vi "lab2_question3.vi"() -> ()   [LabVIEW 2019]
uses:
  <vilib>/Platform/TimedLoop/XDataNode/timing_clust.ctl
  <vilib>/Platform/TimedLoop/XDataNode/nitl_modes.ctl
  <vilib>/Platform/TimedLoop/XDataNode/wakeup.ctl
  <vilib>/Analysis/3filter.llb/Filter Passband Type.ctl
  <vilib>/DAQmx/read.llb/DAQmx Read (Analog DBL 1Chan 1Samp).vi
  <vilib>/DAQmx/create/channels.llb/DAQmx Create Channel (AI-Voltage-Basic).vi
  <vilib>/DAQmx/miscellaneous.llb/DAQmx Fill In Error Info.vi
  <vilib>/platform/TimedLoop/XDataNode/XDataNode.xnode
  <vilib>/Platform/TimedLoop/XDataNode/XDNodeRunTimeDep.lvlib
  <vilib>/ptbypt/NI_PtbyPt.lvlib
  <vilib>/Analysis/NI_AALBase.lvlib
panel:
  out "Position [deg]":dbl(knob) scale=-32.5..32.5
  out "Iteration":i32
  in  "stop":bool
  out "Filtered Signal [V]":dbl
  out "Filtered Signal [V]":dbl(graph)
  in  "low cutoff freq: fl 2":dbl=0.125 format="%0.3f"
  out "Raw Signal [V]":dbl(graph)
  out "Raw Signal [V]":dbl
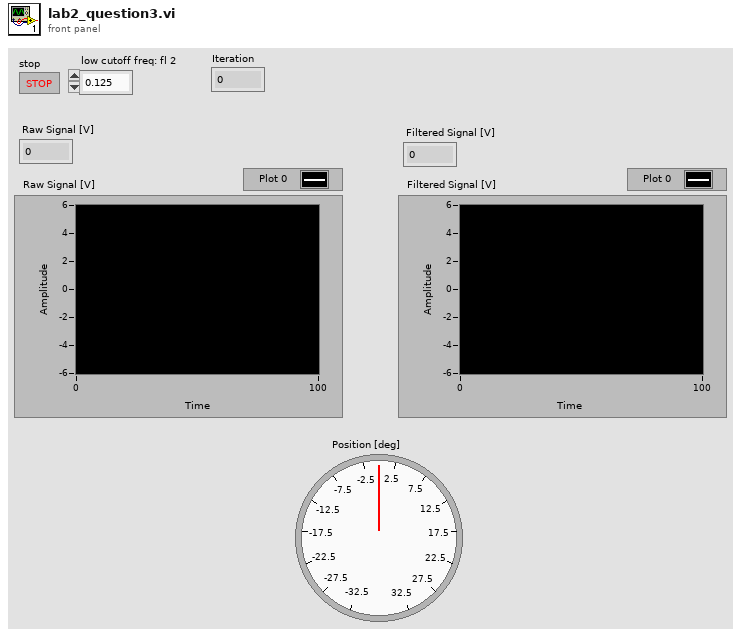
[diagram p1: front panel]
types:
  T1 = typedef "NI_AALBase.lvlib/Filter Passband Type.ctl" = enum32{"Lowpass", "Highpass", "Bandpass", "Bandstop"}
  T2 = typedef "XDNodeRunTimeDep.lvlib/timing_clust.ctl" = cluster{"Expected End [f-1]":u64, "Actual End [f-1]":u64, "Finished Late? [f-1]":bool, "Expected End [i-1]":u64, "Actual End [i-1]":u64, "Finished Late? [i-1]":bool, "Expected Start [i]":u64, "Actual Start [i]":u64, "Expected Start [f]":u64, "Actual Start [f]":u64, "Source Name":string, "Structure Name":string, "Period":i64, "Deadline":i64, "Offset":i64, "Start":i64, "Priority":i32, "Timeout":i32, "Mode":T3, "Wakeup Reason":T4, "Error":errorcluster, "Source Type":string, "Secondary Source Type":string, "Global End Time":u64, "Global Start Time":u64, "Frame Duration":u64, "Iteration Duration":u64, "Assigned CPU":i32, "I/O Scan Engine Mode":u32}
  T3 = typedef "XDNodeRunTimeDep.lvlib/nitl_modes.ctl" = enum32{"No Change", "Process missed periods, maintain original phase", "Discard missed periods, maintain original phase", "Process missed periods, ignore original phase", "Discard missed periods, ignore original phase"}
  T4 = typedef "XDNodeRunTimeDep.lvlib/wakeup.ctl" = enum32{"Normal", "Aborted", "Asynchronous wakeup", "Timing source error", "Timed loop error", "Timeout"}
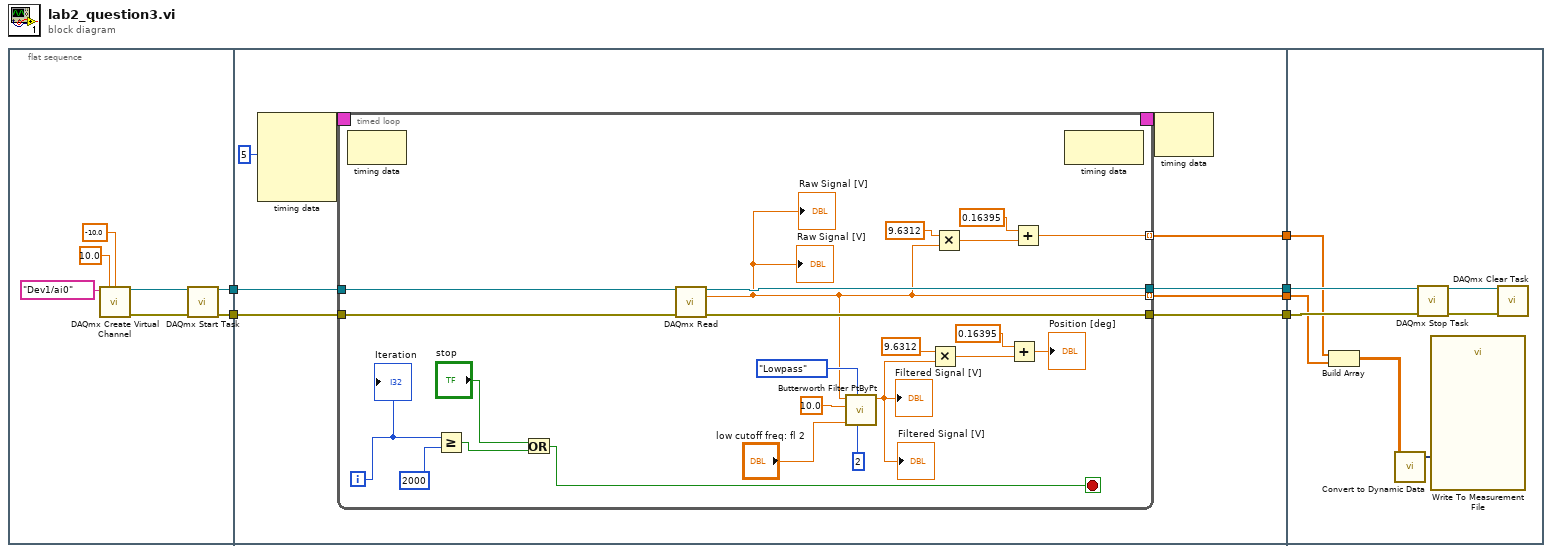
[diagram p0: block diagram]
diagram:
  n1 = flat-sequence {
    tunnel: [w9] -> w6
    tunnel: [w7] -> w3
    tunnel: w6 -> [w20]
    tunnel: [w19] -> w5
    tunnel: [w18] -> w4
    tunnel: w3 -> [w17]
    tunnel: [w16] -> w2
    tunnel: [w14] -> w1
    tunnel: w5 -> [w59]
    tunnel: w4 -> [w54]
    tunnel: w2 -> [w57]
    tunnel: w1 -> [w55]
    frame #0 {
      n2 = call-poly <vilib>:"DAQmx Create Virtual Channel.vi"("maximum value"=10.0, "minimum value"=-10.0, "physical channels"=tag "Dev1/ai0") -> ("task out"=w8:refnum<k21>, "error out"=w10:errorcluster)  [unwired: 11 in]
      n3 = call <vilib>:"DAQmx Start Task.vi"("task/channels in"=w8, "error in"=w10) -> ("task out"=w7:refnum<k21>, "error out"=w9:errorcluster)  [unwired: 12 in]
    }
    frame #1 {
      n4 = node-c288(i64 5 ("Period")) -> (w22:T2)  [unwired: 3 in]
      n5 = timed-loop {
        timing: w22 -> [_]
        timing-out: [_] -> w21
        tunnel: w20 -> [w45]
        tunnel: [w44] -> w19
        tunnel: [w25] -> w18 mode=indexing
        tunnel: w17 -> [w39]
        tunnel: [w38] -> w16
        tunnel: [w23] -> w14 mode=indexing
        i -> [w37]
        stop <- w33 stop-if-true
        n6 = node-c288() -> ()  [unwired: 1 in, 1 out]
        n7 = Greater Or Equal?(x=w37, y=2000) -> (x >= y?=w35:bool)
        n8 = Or(x="stop", y=w35) -> (x .or. y?=w33:bool)
        n9 = call-poly <vilib>:"DAQmx Read.vi"("task/channels in"=w39, "error in"=w45) -> ("task out"=w38:refnum<k21>, "data"=w25:dbl, "error out"=w44:errorcluster)  [unwired: 11 in]
        "Raw Signal [V]" <- w25
        "Raw Signal [V]" <- w25
        n10 = call <vilib>:"Butterworth Filter PtByPt.vi"("order"=2, "filter type"=Filter_Passband_Type."Lowpass", "low cutoff freq: fl"="low cutoff freq: fl 2", "sampling freq: fs"=10.0, "x"=w25) -> ("Filtered x"=w28:dbl)  [unwired: 4 in, 1 out]
        "Filtered Signal [V]" <- w28
        "Filtered Signal [V]" <- w28
        n11 = Multiply(x=9.6312, y=w28) -> (x*y=w31:dbl)
        n12 = Multiply(x=9.6312, y=w25) -> (x*y=w24:dbl)
        n13 = Add(x=0.16395, y=w31) -> (x+y=→"Position [deg]":dbl)
        n14 = Add(x=0.16395, y=w24) -> (x+y=w23:dbl)
        n15 = node-c288() -> ()  [unwired: 1 in, 1 out]
        "Iteration" <- w37
      }
      n16 = node-c288(w21) -> ()  [unwired: 1 out]
    }
    frame #2 {
      n17 = Build Array(w55, w54) -> (w53:dbl[][])
      n18 = call "Convert to Dynamic Data"("2D Array"=w53) -> ("Dynamic Data Type"=w52:dynamicdata)  [unwired: 3 in]
      n19 = call <vilib>:"DAQmx Stop Task.vi"("task/channels in"=w57, "error in"=w59) -> ("task out"=w56:refnum<k21>, "error out"=w58:errorcluster)  [unwired: 12 in]
      n20 = call "Write To Measurement File"("Signals"=w52) -> ()  [unwired: 16 in, 3 out]
      n21 = call <vilib>:"DAQmx Clear Task.vi"("task in"=w56, "error in"=w58) -> ()  [unwired: 13 in, 1 out]
    }
  }
